vi "json_parse_comma.vi"(8 "error in (no error)":errorcluster, 11 "data":string) -> (0 "error out":errorcluster, 3 "remaining data":string)   [LabVIEW 2017]
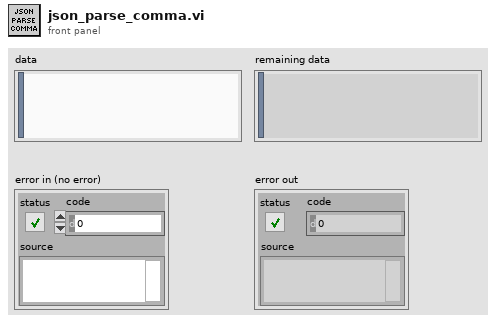
[diagram p1: front panel]
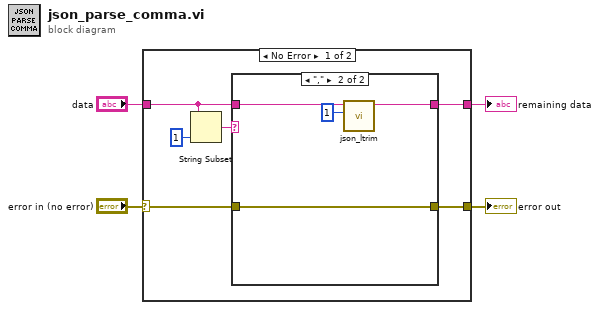
[diagram p0: block diagram]
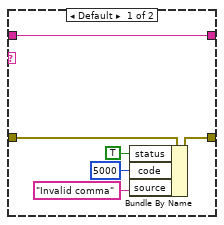
[diagram p2: hidden frame]
diagram:
  n1 = case shown="No Error" "error in (no error)" {
    selector: "error in (no error)" -> [w5 w22]
    tunnel: [w10 w21] -> w4
    tunnel: "data" -> [w9 w21]
    tunnel: [w6 w22] -> w2
    frame No Error {
      n2 = String Subset(string=w9, length (rest)=1 ("length (rest)")) -> (substring=w8:string)  [unwired: 1 in]
      n3 = case shown="\",\"" w8 {
        tunnel: w9 -> [w11 w18]
        tunnel: [w11 w17] -> w10
        tunnel: [w15 w20] -> w6
        tunnel: w5 -> [w16 w20]
        frame Default {
          n4 = Bundle By Name(cluster=w16, "status"=TRUE, "code"=5000, "source"="Invalid comma") -> (w15:errorcluster)
        }
        frame "," {
          n5 = call "json_ltrim.vi"("offset (0)"=1 ("length (rest)"), "data"=w18) -> ("left trim whitespace"=w17:string)  [unwired: 9 in]
        }
      }
    }
    frame Error {
    }
  }
  "remaining data" <- w4
  "error out" <- w2
